vi "Host - Lookup Remote IO ID.vi"(11 "Module ID":u32) -> (0 "RemIO Module Out":refnum<class "RemIO Module.lvclass">, 3 "Module Name":string)   [LabVIEW 2019, in "SEECD System Explorer.lvlib"]
uses:
  SEECD System Explorer.lvlib
  Includes/Modules.lvlibp/RemIO Module/RemIO Module.lvclass
  Includes/Modules.lvlibp/REM-11152/11152.lvclass
  C:/Users/nitest/Desktop/Git/niveristand-scan-engine-ethercat-custom-device/Includes/Modules.lvlibp/RemIO Module/RemIO Module.lvclass
  Includes/Modules.lvlibp/REM-11115/11115.lvclass
  Includes/Modules.lvlibp/REM-11154/11154.lvclass
  Includes/Modules.lvlibp/REM-11175/11175.lvclass
  Includes/Modules.lvlibp/REM-11178/11178.lvclass
  Includes/Modules.lvlibp/REM-11102/11102.lvclass
  Includes/Modules.lvlibp/REM-11100/11100.lvclass
  Includes/Modules.lvlibp/REM-11120/11120.lvclass
panel:
  out "Number of Outputs":u32
  out "Number of Inputs":u32
  out "Module Pdo Group":string
  out "Module Class":string
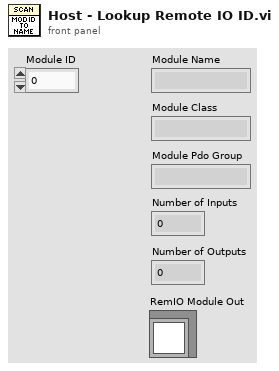
[diagram p1: front panel]
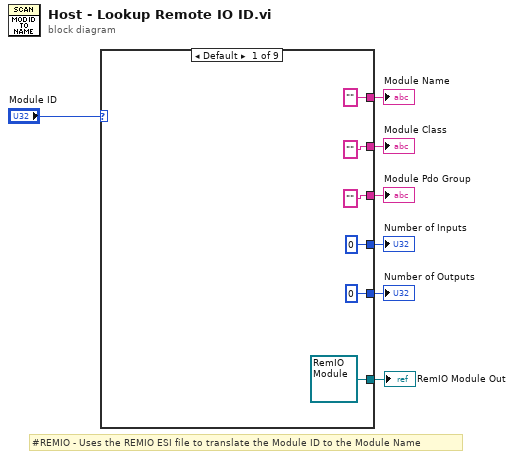
[diagram p0: block diagram]
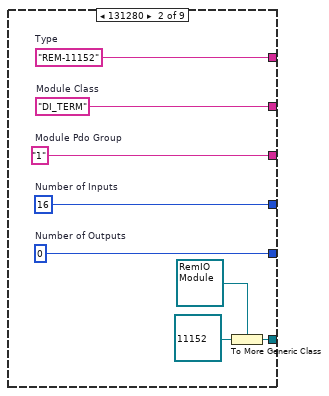
[diagram p2: hidden frame]
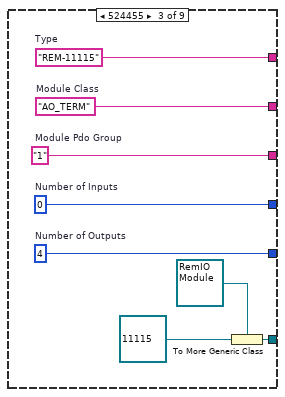
[diagram p3: hidden frame]
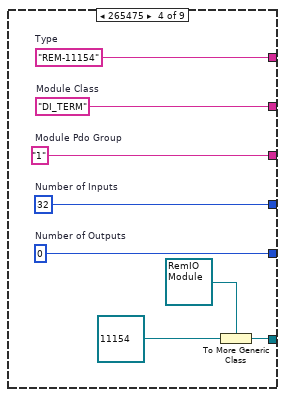
[diagram p4: hidden frame]
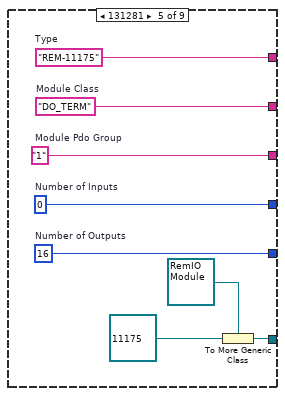
[diagram p5: hidden frame]
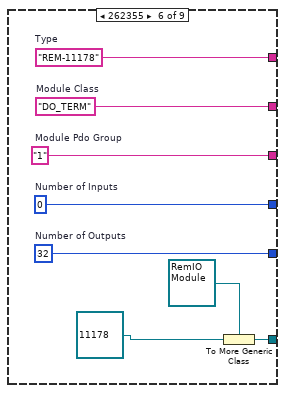
[diagram p6: hidden frame]
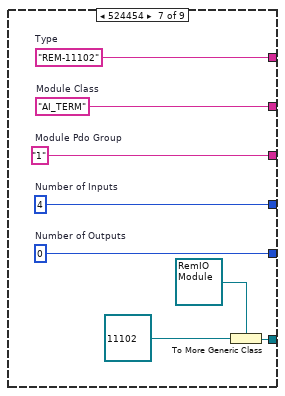
[diagram p7: hidden frame]
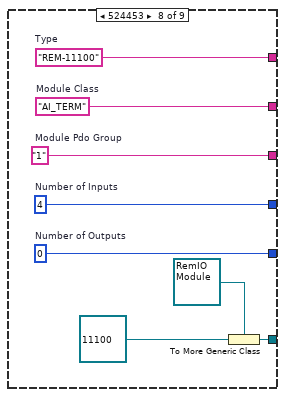
[diagram p8: hidden frame]
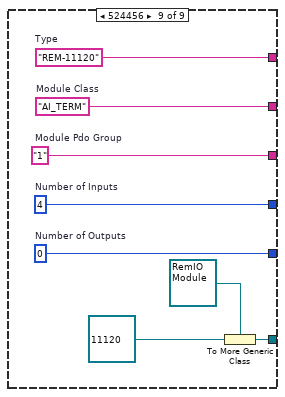
[diagram p9: hidden frame]
diagram:
  # "#REMIO - Uses the REMIO ESI file to translate the Module ID to the Module Name"
  n1 = case shown="Default" "Module ID" {
    tunnel: ["" ("Type") w21 w29 w37 w45 w53 w61 w69 w77] -> w6
    tunnel: ["" ("Module Class") w20 w28 w36 w44 w52 w60 w68 w76] -> w5
    tunnel: ["" ("Module Pdo Group") w19 w27 w35 w43 w51 w59 w67 w75] -> w4
    tunnel: [u32 0 ("Number of Inputs") w18 w26 w34 w42 w50 w58 w66 w74] -> w3
    tunnel: [u32 0 ("Number of Outputs") w17 w25 w33 w41 w49 w57 w65 w73] -> w2
    tunnel: [refnum<class "RemIO Module.lvclass"> refnum ("RemIO Module Out") w14 w23 w30 w39 w47 w55 w63 w71] -> w1
    frame Default {
    }
    frame 131280 {
      w17 = u32 0  # Number of Outputs
      w18 = u32 16  # Number of Inputs
      w19 = "1"  # Module Pdo Group
      w20 = "DI_TERM"  # Module Class
      w21 = "REM-11152"  # Type
      n2 = To More Generic Class(target class=refnum<class "RemIO Module.lvclass"> refnum ("RemIO Module Out"), reference=refnum<class "11152.lvclass"> refnum ("Modules.lvlibp:11152.lvclass")) -> (generic class reference=w14:refnum<class "RemIO Module.lvclass">)
    }
    frame 524455 {
      w25 = u32 4  # Number of Outputs
      w26 = u32 0  # Number of Inputs
      w27 = "1"  # Module Pdo Group
      w28 = "AO_TERM"  # Module Class
      w29 = "REM-11115"  # Type
      n3 = To More Generic Class(target class=refnum<class "RemIO Module.lvclass"> refnum ("RemIO Module Out"), reference=refnum<class "11115.lvclass"> refnum ("Modules.lvlibp:11115.lvclass")) -> (generic class reference=w23:refnum<class "RemIO Module.lvclass">)
    }
    frame 265475 {
      w33 = u32 0  # Number of Outputs
      w34 = u32 32  # Number of Inputs
      w35 = "1"  # Module Pdo Group
      w36 = "DI_TERM"  # Module Class
      w37 = "REM-11154"  # Type
      n4 = To More Generic Class(target class=refnum<class "RemIO Module.lvclass"> refnum ("RemIO Module Out"), reference=refnum<class "11154.lvclass"> refnum ("Modules.lvlibp:11154.lvclass")) -> (generic class reference=w30:refnum<class "RemIO Module.lvclass">)
    }
    frame 131281 {
      w41 = u32 16  # Number of Outputs
      w42 = u32 0  # Number of Inputs
      w43 = "1"  # Module Pdo Group
      w44 = "DO_TERM"  # Module Class
      w45 = "REM-11175"  # Type
      n5 = To More Generic Class(target class=refnum<class "RemIO Module.lvclass"> refnum ("RemIO Module Out"), reference=refnum<class "11175.lvclass"> refnum ("Modules.lvlibp:11175.lvclass")) -> (generic class reference=w39:refnum<class "RemIO Module.lvclass">)
    }
    frame 262355 {
      w49 = u32 32  # Number of Outputs
      w50 = u32 0  # Number of Inputs
      w51 = "1"  # Module Pdo Group
      w52 = "DO_TERM"  # Module Class
      w53 = "REM-11178"  # Type
      n6 = To More Generic Class(target class=refnum<class "RemIO Module.lvclass"> refnum ("RemIO Module Out"), reference=refnum<class "11178.lvclass"> refnum ("Modules.lvlibp:11178.lvclass")) -> (generic class reference=w47:refnum<class "RemIO Module.lvclass">)
    }
    frame 524454 {
      w57 = u32 0  # Number of Outputs
      w58 = u32 4  # Number of Inputs
      w59 = "1"  # Module Pdo Group
      w60 = "AI_TERM"  # Module Class
      w61 = "REM-11102"  # Type
      n7 = To More Generic Class(target class=refnum<class "RemIO Module.lvclass"> refnum ("RemIO Module Out"), reference=refnum<class "11102.lvclass"> refnum ("Modules.lvlibp:11102.lvclass")) -> (generic class reference=w55:refnum<class "RemIO Module.lvclass">)
    }
    frame 524453 {
      w65 = u32 0  # Number of Outputs
      w66 = u32 4  # Number of Inputs
      w67 = "1"  # Module Pdo Group
      w68 = "AI_TERM"  # Module Class
      w69 = "REM-11100"  # Type
      n8 = To More Generic Class(target class=refnum<class "RemIO Module.lvclass"> refnum ("RemIO Module Out"), reference=refnum<class "11100.lvclass"> refnum ("Modules.lvlibp:11100.lvclass")) -> (generic class reference=w63:refnum<class "RemIO Module.lvclass">)
    }
    frame 524456 {
      w73 = u32 0  # Number of Outputs
      w74 = u32 4  # Number of Inputs
      w75 = "1"  # Module Pdo Group
      w76 = "AI_TERM"  # Module Class
      w77 = "REM-11120"  # Type
      n9 = To More Generic Class(target class=refnum<class "RemIO Module.lvclass"> refnum ("RemIO Module Out"), reference=refnum<class "11120.lvclass"> refnum ("Modules.lvlibp:11120.lvclass")) -> (generic class reference=w71:refnum<class "RemIO Module.lvclass">)
    }
  }
  "Module Name" <- w6
  "Module Class" <- w5
  "Module Pdo Group" <- w4
  "Number of Inputs" <- w3
  "Number of Outputs" <- w2
  "RemIO Module Out" <- w1
